vi "Update.vi"(8 "error in (no error)":errorcluster caption="entrée d'erreur (pas d'erreur)", 11 "Level Controller en entrée":refnum<class "Level Controller.lvclass">) -> (0 "error out":errorcluster caption="sortie d'erreur", 3 "Level Controller en sortie":refnum<class "Level Controller.lvclass">)   [LabVIEW 2015, in "Level Controller.lvlib" / "Level Controller.lvclass"]
uses:
  Level Controller.lvclass
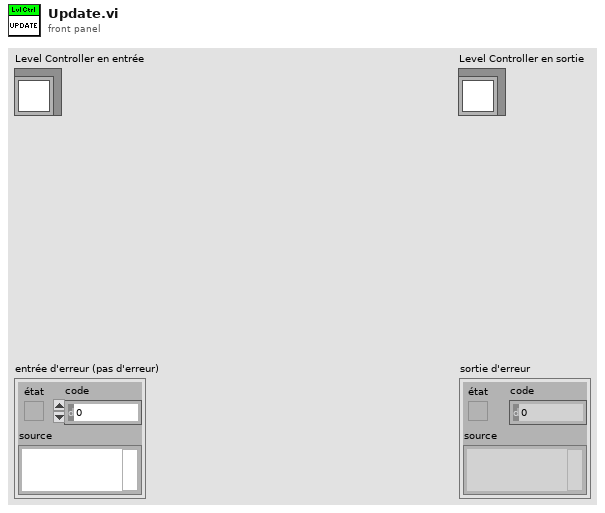
[diagram p1: front panel]
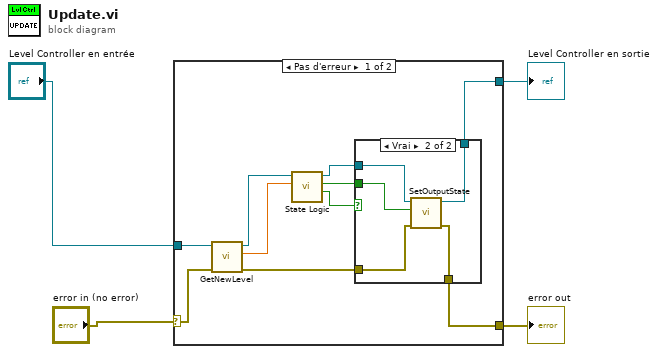
[diagram p0: block diagram]
diagram:
  n1 = case shown="Pas d'erreur" "error in (no error)" {
    selector: "error in (no error)" -> [w14 w22]
    tunnel: "Level Controller en entrée" -> [w13 w23]
    tunnel: [w6 w23] -> w2
    tunnel: [w5 w22] -> w1
    frame No Error {
      n2 = call-dynamic "GetNewLevel.vi"("error in (no error)"=w14, "Level Controller en entrée"=w13) -> ("error out"=w7:errorcluster, "Level"=w11:dbl, "Level Controller en sortie"=w12:refnum<class "Level Controller.lvclass">)  [unwired: 7 in]
      n3 = call "State Logic.vi"("Level"=w11, "Level Controller in"=w12) -> ("State Changed"=w10:bool, "Output State"=w9:bool, "Level Controller out"=w8:refnum<class "Level Controller.lvclass">)  [unwired: 7 in]
      n4 = case shown="Vrai" w10 {
        tunnel: w9 -> [_ w21]
        tunnel: w8 -> [w16 w20]
        tunnel: w7 -> [w15 w19]
        tunnel: [w16 w18] -> w6
        tunnel: [w15 w17] -> w5
        frame False {
        }
        frame True {
          n5 = call-dynamic "SetOutputState.vi"("error in (no error)"=w19, "Output State"=w21, "Level Controller en entrée"=w20) -> ("error out"=w17:errorcluster, "Level Controller en sortie"=w18:refnum<class "Level Controller.lvclass">)  [unwired: 7 in]
        }
      }
    }
    frame Error {
    }
  }
  "error out" <- w1
  "Level Controller en sortie" <- w2
